vi "Conversor.vi"() -> ()   [LabVIEW 2016]
panel:
  in  "D":bool
  in  "C":bool
  in  "B":bool
  in  "A":bool
  out "C0":bool
  out "C1":bool
  out "C2":bool
  out "C3":bool
  out "C4":bool
  out "B0":bool
  out "B1":bool
  out "B2":bool
  out "B3":bool
  out "B4":bool
  out "A0":bool
  out "A1":bool
  out "A2":bool
  out "A3":bool
  # "Código Gray"
  # "BCD"
  # "XA-3"
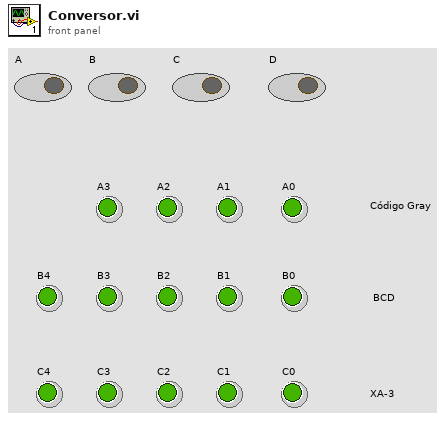
[diagram p1: front panel]
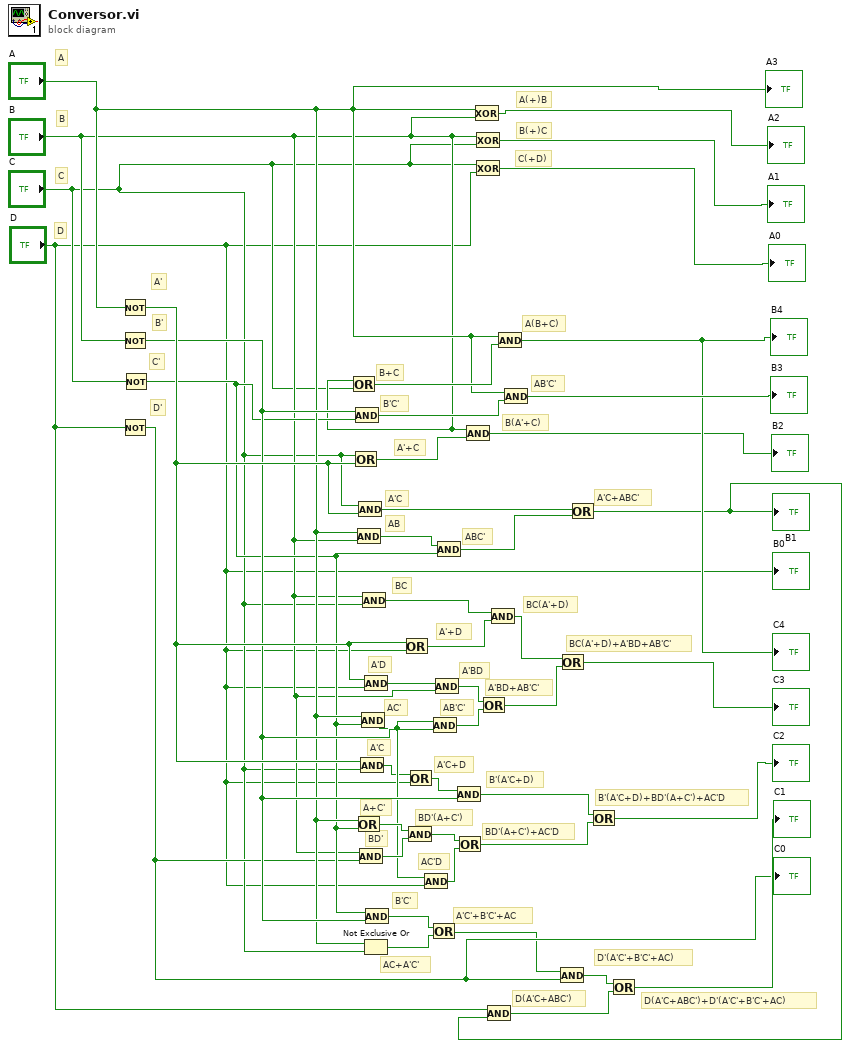
[diagram p0: block diagram]
diagram:
  # "AC'D"
  # "A'BD+AB'C'"
  # "AB'C'"
  # "A'BD"
  # "D(A'C+ABC')+D'(A'C'+B'C'+AC)"
  # "D(A'C+ABC')"
  # "D'(A'C'+B'C'+AC)"
  # "A'C'+B'C'+AC"
  # "AC+A'C'"
  # "B'C'"
  # "B'(A'C+D)+BD'(A+C')+AC'D"
  # "BD'(A+C')+AC'D"
  # "BD'"
  # "BD'(A+C')"
  # "A+C'"
  # "B'(A'C+D)"
  # "A'C+D"
  # "A'C"
  # "BC(A'+D)+A'BD+AB'C'"
  # "A'D"
  # "AC'"
  # "BC(A'+D)"
  # "A'+D"
  # "BC"
  # "A'C+ABC'"
  # "A'C"
  # "ABC'"
  # "AB"
  # "B(A'+C)"
  # "A'+C"
  # "AB'C'"
  # "B'C'"
  # "A(B+C)"
  # "B+C"
  # "D'"
  # "C'"
  # "B'"
  # "A'"
  # "C(+D)"
  # "B(+)C"
  # "A(+)B"
  # "D"
  # "C"
  # "B"
  # "A"
  n1 = Not(x="A") -> (.not. x?=w21:bool)
  n2 = Not(x="B") -> (.not. x?=w16:bool)
  n3 = Not(x="D") -> (.not. x?=w9:bool)
  "C0" <- w9
  n4 = Not(x="C") -> (.not. x?=w11:bool)
  n5 = Or(x="B", y="C") -> (x .or. y?=w41:bool)
  n6 = Or(x="C", y=w21) -> (x .or. y?=w38:bool)
  n7 = And(x=w16, y=w11) -> (x .and. y?=w39:bool)
  n8 = And(x="A", y="B") -> (x .and. y?=w36:bool)
  n9 = Or(x="A", y=w11) -> (x .or. y?=w14:bool)
  n10 = And(x="C", y=w21) -> (x .and. y?=w34:bool)
  n11 = And(x="B", y=w9) -> (x .and. y?=w15:bool)
  n12 = And(x=w21, y="C") -> (x .and. y?=w5:bool)
  n13 = And(x="A", y=w11) -> (x .and. y?=w8:bool)
  n14 = And(x="B", y="C") -> (x .and. y?=w33:bool)
  n15 = And(x=w21, y="D") -> (x .and. y?=w17:bool)
  n16 = Not Exclusive Or(1:"C", 2:"A") -> (0:w26:bool)
  n17 = And(x=w11, y=w16) -> (x .and. y?=w27:bool)
  n18 = Or(x=w21, y="D") -> (x .or. y?=w32:bool)
  n19 = And(x=w14, y=w15) -> (x .and. y?=w13:bool)
  n20 = Or(x=w5, y="D") -> (x .or. y?=w29:bool)
  n21 = And(x=w8, y="D") -> (x .and. y?=w6:bool)
  n22 = Or(x=w27, y=w26) -> (x .or. y?=w2:bool)
  n23 = And(x=w8, y=w16) -> (x .and. y?=w19:bool)
  n24 = And(x=w17, y="B") -> (x .and. y?=w20:bool)
  n25 = And(x=w36, y=w11) -> (x .and. y?=w35:bool)
  n26 = And(x=w29, y=w16) -> (x .and. y?=w28:bool)
  n27 = Or(x=w13, y=w6) -> (x .or. y?=w7:bool)
  n28 = And(x="B", y=w38) -> (x .and. y?=→"B2":bool)
  n29 = Exclusive Or(1:"B", 2:"A") -> (0:→"A2":bool)
  n30 = Exclusive Or(1:"C", 2:"B") -> (0:→"A1":bool)
  n31 = Exclusive Or(1:"D", 2:"C") -> (0:→"A0":bool)
  n32 = Or(x=w20, y=w19) -> (x .or. y?=w18:bool)
  n33 = And(x=w33, y=w32) -> (x .and. y?=w31:bool)
  n34 = And(x="A", y=w41) -> (x .and. y?=→"B4" →"C4":bool)
  n35 = And(x="A", y=w39) -> (x .and. y?=→"B3":bool)
  n36 = And(x=w2, y=w9) -> (x .and. y?=w23:bool)
  n37 = Or(x=w31, y=w18) -> (x .or. y?=→"C3":bool)
  n38 = Or(x=w34, y=w35) -> (x .or. y?=w24:bool)
  "B1" <- w24
  n39 = And(x="D", y=w24) -> (x .and. y?=w25:bool)
  n40 = Or(x=w28, y=w7) -> (x .or. y?=→"C2":bool)
  n41 = Or(x=w23, y=w25) -> (x .or. y?=→"C1":bool)
  "A3" <- "A"
  "B0" <- "D"
